vi "NI6071E_RT_Main.vi"(9 "Port":u16=6341) -> ()   [LabVIEW 2009]
uses:
  NI6071ECommand.ctl
  NI6071ECommandCluster.ctl
  NI6071EConfig.ctl
  NI6071EStart.ctl
  NI6071ERead.ctl
  <vilib>/Utility/error.llb/DialogType.ctl
  NI6071E.lvlib
panel:
  out "remote address":string
  in  "NI6071E DAQ Read":T1={"time limit in sec (-1:auto calculate)"=-1.0, "number of scans to read (-1:all)"=-1} {"time limit in sec (-1:auto calculate)" format="%0.2f"}
  in  "NI6071E DAQ Start":T2={"scan rate (40000 scans/sec)"=1000.0, "trigger type (analog)"=enum."no trigger", "edge or slope \n(rising)"=enum."no change", "number of buffers to acquire (1)"=1, "analog chan (PFI0) & level (2.00)"={"trigger channel (empty)"="", "level (0.0)"=0.0}, "[additional trig params]"={"hysteresis (0.0)"=-1.0, "coupling (no change:0)"=enum."no change", "delay (0 sec)"=0.0, "skip count (0)"=0, "time limit (0 sec)"=0.0}} {"[additional trig params]"."time limit (0 sec)" format="%0.2f"; "[additional trig params]"."delay (0 sec)" format="%0.2f"; "[additional trig params]"."hysteresis (0.0)" format="%0.2f"; "analog chan (PFI0) & level (2.00)"."level (0.0)" format="%0.2f"; "scan rate (40000 scans/sec)" format="%0.2f"}
  out "NI6071E DAQ Config":T3={"device (1)"=1, "channels (0)"=["0"], "buffer size (1000 scans)"=1000, "[number of buffers] (1)"=1, "measurement mode structure"={"measurement mode"=0, "reserved"=0}, "input limits (no change)"=[], "coupling & input config (no change:0)"=[]} {"measurement mode structure"."measurement mode" items=["no change", "Volts", "Volts RMS", "Ohms", "Diode", "4-wire ohms", "Current", "Current RMS"]; "coupling & input config (no change:0)"."input config (no change:0)" items=["no change", "differential", "ref. single-ended", "non-ref. single-ended", "4-wire"]; "input limits (no change)"."low limit (0.0)" format="%0.2f"; "input limits (no change)"."high limit (0.0)" format="%0.2f"}
  in  "NI6071E Config Default":T3={"device (1)"=1, "channels (0)"=["0"], "buffer size (1000 scans)"=1000, "[number of buffers] (1)"=1, "measurement mode structure"={"measurement mode"=0, "reserved"=0}, "input limits (no change)"=[], "coupling & input config (no change:0)"=[]} {"measurement mode structure"."measurement mode" items=["no change", "Volts", "Volts RMS", "Ohms", "Diode", "4-wire ohms", "Current", "Current RMS"]; "coupling & input config (no change:0)"."input config (no change:0)" items=["no change", "differential", "ref. single-ended", "non-ref. single-ended", "4-wire"]; "input limits (no change)"."low limit (0.0)" format="%0.2f"; "input limits (no change)"."high limit (0.0)" format="%0.2f"}
  in  "taskID in":u32 format="%x"
  out "Error string":string
  in  "NI6071E Command Cluster":T4
  out "Measurement":waveform(dbl)[](graph)
  out "NI6071E Command":T5=enum."ConfigureDAQ"
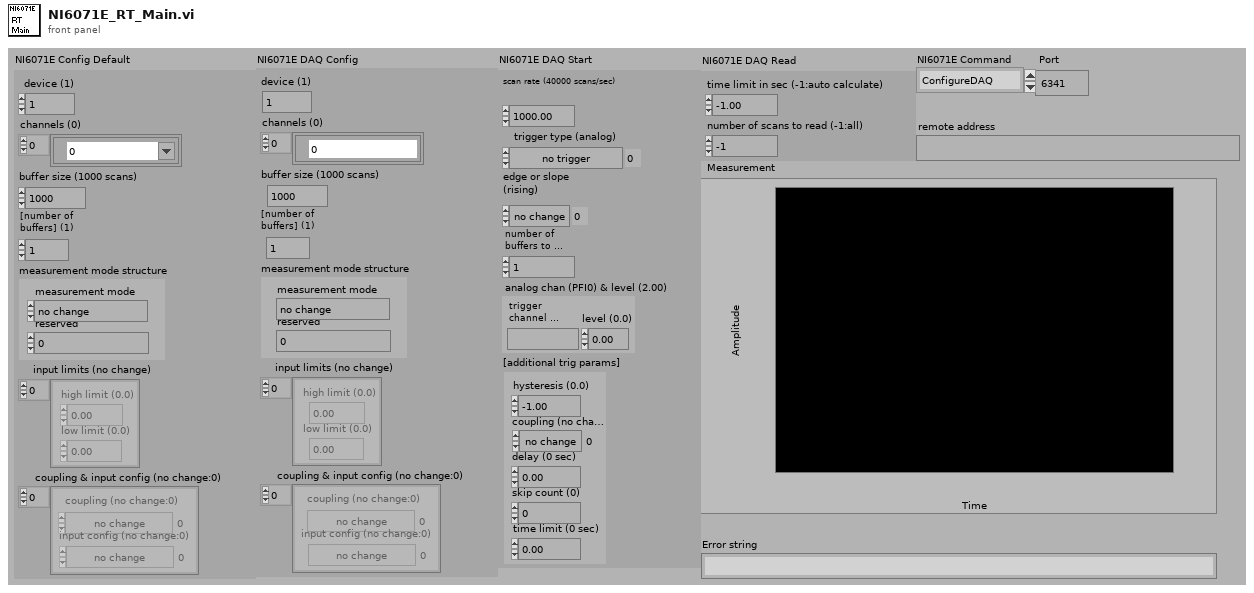
[diagram p1: front panel]
types:
  T1 = typedef "NI6071E.lvlib/NI6071ERead.ctl" = cluster{"time limit in sec (-1:auto calculate)":sgl, "number of scans to read (-1:all)":i32}
  T2 = typedef "NI6071E.lvlib/NI6071EStart.ctl" = cluster{"scan rate (40000 scans/sec)":sgl, "trigger type (analog)":enum16{"no trigger", "analog", "digital A", "digital A & B", "scan clock gate"}, "edge or slope \n(rising)":enum16{"no change", "rising", "falling"}, "number of buffers to acquire (1)":i32, "analog chan (PFI0) & level (2.00)":cluster{"trigger channel (empty)":string, "level (0.0)":sgl}, "[additional trig params]":cluster{"hysteresis (0.0)":sgl, "coupling (no change:0)":enum16{"no change", "DC", "AC"}, "delay (0 sec)":sgl, "skip count (0)":i32, "time limit (0 sec)":sgl}}
  T3 = typedef "NI6071E.lvlib/NI6071EConfig.ctl" = cluster{"device (1)":i16, "channels (0)":tag[], "buffer size (1000 scans)":i32, "[number of buffers] (1)":i32, "measurement mode structure":cluster{"measurement mode":u16, "reserved":u32}, "input limits (no change)":cluster{"high limit (0.0)":sgl, "low limit (0.0)":sgl}[], "coupling & input config (no change:0)":cluster{"coupling (no change:0)":enum16{"no change", "DC", "AC", "GND", "internal ref."}, "input config (no change:0)":u16}[]}
  T4 = typedef "NI6071E.lvlib/NI6071ECommandCluster.ctl" = cluster{"Command":string, "Data":string, "error out":errorcluster}
  T5 = typedef "NI6071E.lvlib/NI6071ECommand.ctl" = enum16{"Ping", "Reset", "ConfigureDAQ", "StartDAQ", "StopDAQ", "GetDAQStatus", "ReadData", "SaveData", "CloseConnection"}
  T6 = typedef "DialogType.ctl" = u16
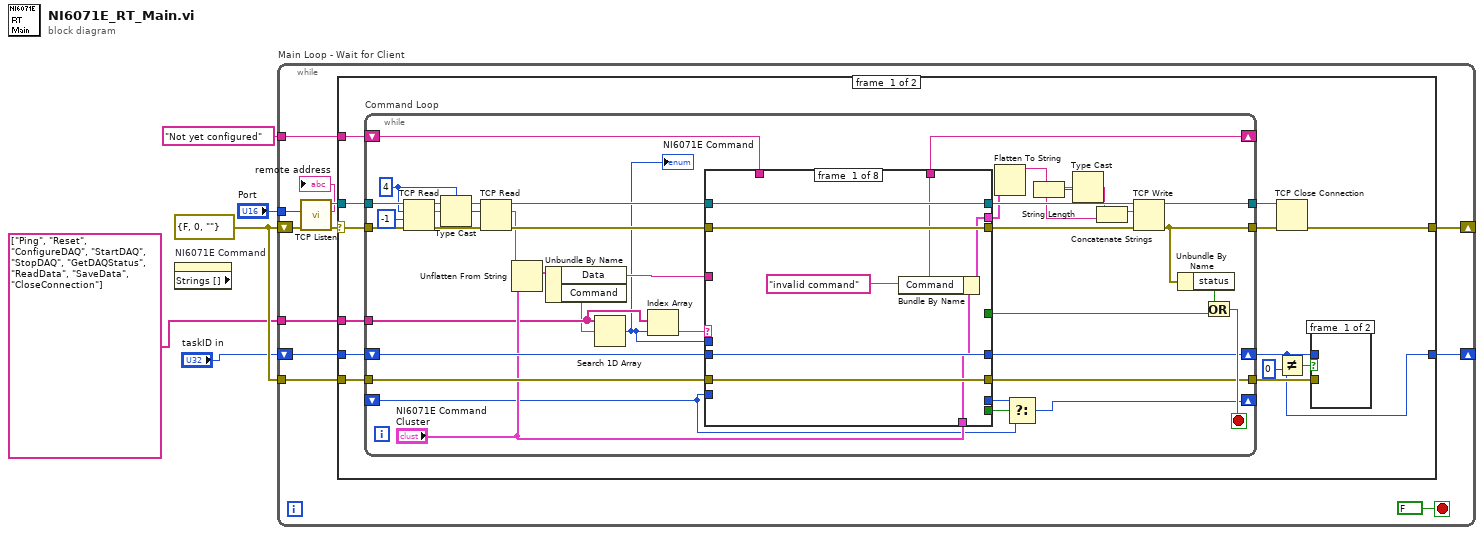
[diagram p0: block diagram]
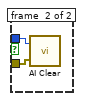
[diagram p2: hidden frame]
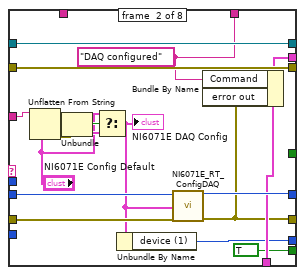
[diagram p3: hidden frame]
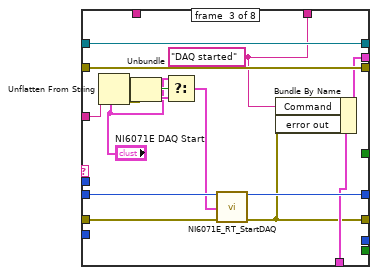
[diagram p4: hidden frame]
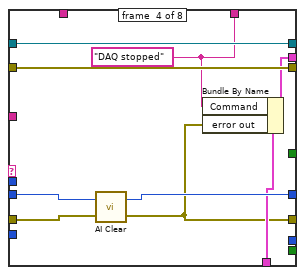
[diagram p5: hidden frame]
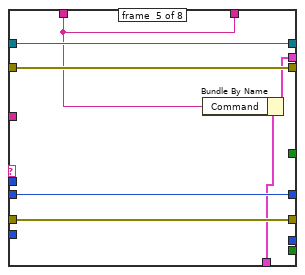
[diagram p6: hidden frame]
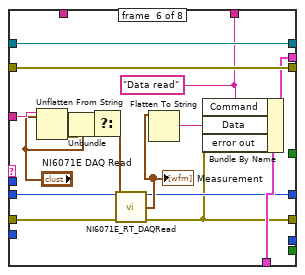
[diagram p7: hidden frame]
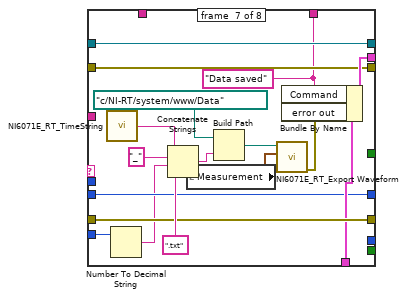
[diagram p8: hidden frame]
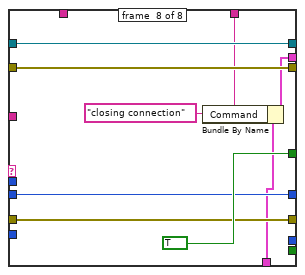
[diagram p9: hidden frame]
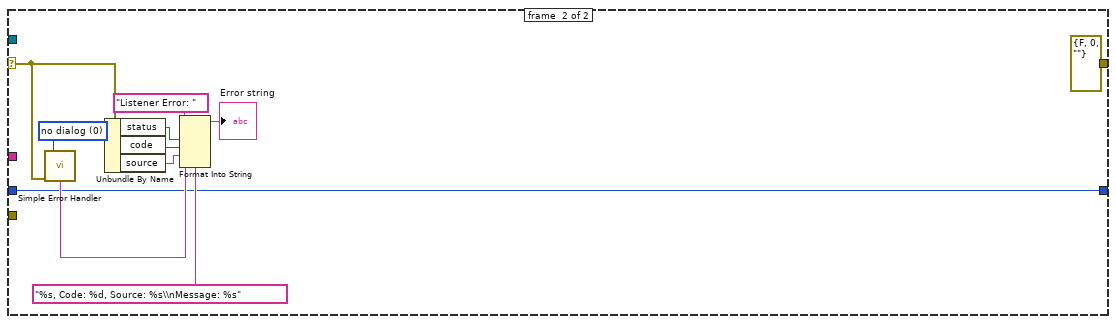
[diagram p10: hidden frame]
diagram:
  w5 = errorcluster {"status"=FALSE, "code"=0, "source"=""} ("error out")
  n1 = property on="NI6071E Command" class="Enum (strict)" props=["Strings []"]() -> ()  [unwired: 2 in, 3 out]
  n2 = while "Main Loop - Wait for Client" {
    tunnel: "Port" -> [w17]
    shift-right: [w12] -> _
    shift-left: w5 -> [w13]
    tunnel: string[] ["Ping", "Reset", "ConfigureDAQ", "StartDAQ", "StopDAQ", "GetDAQStatus", "ReadData", "SaveData", "CloseConnection"] ("Strings []") -> [w11]
    shift-right: [w9] -> _
    shift-left: "taskID in" -> [w10]
    tunnel: w5 -> [w8]
    tunnel: "Not yet configured" -> [w7]
    stop <- FALSE stop-if-true
    n3 = call <vilib>:"TCP Listen.vi"("error in (no error)"=w13, "port"=w17) -> ("error out"=w16:errorcluster, "remote address"=→"remote address":string, "connection ID"=w14:refnum<k5>)  [unwired: 6 in, 1 out]
    n4 = case shown="No Error" w16 {
      selector: w16 -> [w29 w173]
      tunnel: w14 -> [w30 _]
      tunnel: [w27 errorcluster {"status"=FALSE, "code"=0, "source"=""} ("error out")] -> w12
      tunnel: w11 -> [w25 _]
      tunnel: w10 -> [w24 w171]
      tunnel: [w19 w171] -> w9
      tunnel: w8 -> [w20 _]
      tunnel: w7 -> [w18 _]
      frame #0 {
        w19 = u32 0 ("taskID in")
        n5 = while "Command Loop" {
          tunnel: w30 -> [w72]
          tunnel: w29 -> [w71]
          tunnel: [w57] -> w28
          tunnel: [w58] -> w26
          tunnel: w25 -> [w36]
          tunnel: w20 -> [w46]
          tunnel: [w47] -> w21
          shift-right: [w51] -> w22
          shift-left: w24 -> [w52]
          shift-right: [w42] -> _
          shift-left: w18 -> [w41]
          shift-right: [w38] -> _
          shift-left: _ -> [w37]
          stop <- w61 stop-if-true
          w68 = 4 ("bytes to read")
          n6 = TCP Read(connection ID=w72, bytes to read=w68, error in (no error)=w71, 9:-1 ("timeout ms (25000)")) -> (connection ID out=w67:refnum<k5>, data out=w69:string, error out=w66:errorcluster)  [unwired: 1 in]
          n7 = Type Cast(type=w68, x=w69) -> (*(type *) &x=w53:i32)
          n8 = TCP Read(connection ID=w67, bytes to read=w53, error in (no error)=w66) -> (connection ID out=w64:refnum<k5>, data out=w49:string, error out=w65:errorcluster)  [unwired: 2 in]
          n9 = Unflatten From String(type="NI6071E Command Cluster", binary string=w49) -> (value=w50:T4)  [unwired: 3 in, 2 out]
          n10 = Unbundle By Name(w50) -> ("Data"=w48:string, "Command"=w34:string)
          n11 = Search 1D Array(1D array=w36, element=w34) -> (index of element=w35:i32)  [unwired: 1 in]
          "NI6071E Command" <- w35
          n12 = Index Array(array=w36, index=w35) -> (element=w33:string)
          n13 = case shown="\"ConfigureDAQ\"" w33 {
            tunnel: [_ _ _ _ _ _ _ TRUE] -> w62
            tunnel: w65 -> [w78 w92 w107 w117 w126 w143 w150 w167]
            tunnel: w64 -> [w79 w96 w111 w120 w127 w144 w161 w168]
            tunnel: [w79 w96 w111 w120 w127 w144 w161 w168] -> w59
            tunnel: [w78 w92 w107 w117 w126 w143 w150 w167] -> w60
            tunnel: [w74 w86 w105 w114 w122 w138 w152 w163] -> w44
            tunnel: w52 -> [w77 w91 w110 w119 w125 w129 w147 w166]
            tunnel: [w77 w90 w109 w118 w125 w134 w147 w166] -> w51
            tunnel: w48 -> [_ w95 w100 _ _ w140 _ _]
            tunnel: [w76 w85 w104 w113 w124 w133 w154 w165] -> w47
            tunnel: w46 -> [w76 w89 w108 w116 w124 w132 w154 w165]
            tunnel: "NI6071E Command Cluster" -> [w75 w87 w106 w115 w123 w137 w153 w164]
            tunnel: [w73 w84 w98 w112 w121 w136 w149 w162] -> w42
            tunnel: w41 -> [_ _ _ _ w121 _ _ _]
            tunnel: [_ w82 _ _ _ _ _ _] -> w40
            tunnel: [_ TRUE _ _ _ _ _ _] -> w39
            tunnel: w37 -> [_ _ _ _ _ _ w146 _]
            tunnel: w35 -> [_ _ _ _ _ _ _ _]
            frame #0 {
              w73 = "invalid command"
              n14 = Bundle By Name(cluster=w75, "Command"=w73) -> (w74:T4)
            }
            frame #1 {
              w84 = "DAQ configured"
              n15 = Unflatten From String(type="NI6071E Config Default", binary string=w95) -> (value=w93:T3, error out=w80:errorcluster)  [unwired: 3 in, 1 out]
              n16 = Unbundle(w80) -> ("status"=w94:bool)  [unwired: 2 out]
              n17 = Select(t="NI6071E Config Default", s=w94, f=w93) -> (s? t:f=w83:T3)
              "NI6071E DAQ Config" <- w83
              n18 = Unbundle By Name(w83) -> ("device (1)"=w82:i16)
              n19 = call "NI6071E_RT_ConfigDAQ.vi"("taskID in"=w91, "NI6071E DAQ Config"=w83, "error in (no error)"=w89) -> ("taskID out"=w90:u32, "error out"=w85:errorcluster)  [unwired: 10 in, 1 out]
              n20 = Bundle By Name(cluster=w87, "Command"=w84, "error out"=w85) -> (w86:T4)
            }
            frame #2 {
              w98 = "DAQ started"
              n21 = Unflatten From String(type="NI6071E DAQ Start", binary string=w100) -> (value=w102:T2, error out=w97:errorcluster)  [unwired: 3 in, 1 out]
              n22 = Unbundle(w97) -> ("status"=w103:bool)  [unwired: 2 out]
              n23 = Select(t="NI6071E DAQ Start", s=w103, f=w102) -> (s? t:f=w99:T2)
              n24 = call "NI6071E_RT_StartDAQ.vi"("taskID in"=w110, "NI6071E DAQ Start"=w99, "error in"=w108) -> ("taskID out"=w109:u32, "error out"=w104:errorcluster)  [unwired: 11 in]
              n25 = Bundle By Name(cluster=w106, "Command"=w98, "error out"=w104) -> (w105:T4)
            }
            frame #3 {
              w112 = "DAQ stopped"
              n26 = call <vilib>:"AI Clear.vi"("error in (no error)"=w116, "taskID in"=w119) -> ("error out"=w113:errorcluster, "taskID out"=w118:u32)  [unwired: 4 in]
              n27 = Bundle By Name(cluster=w115, "Command"=w112, "error out"=w113) -> (w114:T4)
            }
            frame #4 {
              n28 = Bundle By Name(cluster=w123, "Command"=w121) -> (w122:T4)
            }
            frame #5 {
              w136 = "Data read"
              n29 = Unflatten From String(type="NI6071E DAQ Read", binary string=w140) -> (value=w141:T1, error out=w128:errorcluster)  [unwired: 3 in, 1 out]
              n30 = Unbundle(w128) -> ("status"=w142:bool)  [unwired: 2 out]
              n31 = Select(t="NI6071E DAQ Read", s=w142, f=w141) -> (s? t:f=w130:T1)
              n32 = call "NI6071E_RT_DAQRead.vi"("taskID in"=w129, "NI6071E Read"=w130, "error in"=w132) -> ("taskID out"=w134:u32, "Measurement"=w135:waveform(dbl)[], "error out"=w133:errorcluster)  [unwired: 10 in]
              "Measurement" <- w135
              n33 = Flatten To String(anything=w135) -> (data string=w139:string)  [unwired: 3 in, 2 out]
              n34 = Bundle By Name(cluster=w137, "Command"=w136, "Data"=w139, "error out"=w133) -> (w138:T4)
            }
            frame #6 {
              w149 = "Data saved"
              n35 = call "NI6071E_RT_TimeString.vi"() -> ("date/time string"=w157:string)
              n36 = Number To Decimal String(number=w146) -> (decimal integer string=w145:string)  [unwired: 1 in]
              n37 = Concatenate Strings(w157, "_" ("string"), w145, ".txt" ("string")) -> (w155:string)
              n38 = local read "Measurement"() -> (w160:waveform(dbl)[])
              n39 = Build Path(base path=path "c:/NI-RT/system/www/Data" ("file path (dialog if empty)"), name or relative path=w155) -> (appended path=w158:path)
              n40 = call "NI6071E_RT_Export Waveform.vi"("Waveforms"=w160, "file path (dialog if empty)"=w158) -> ("error out"=w151:errorcluster)  [unwired: 8 in, 1 out]
              n41 = Bundle By Name(cluster=w153, "Command"=w149, "error out"=w151) -> (w152:T4)
            }
            frame #7 {
              w162 = "closing connection"
              n42 = Bundle By Name(cluster=w164, "Command"=w162) -> (w163:T4)
            }
          }
          n43 = Flatten To String(anything=w44) -> (data string=w45:string)  [unwired: 3 in, 2 out]
          n44 = Select(t=w40, s=w39, f=w37) -> (s? t:f=w38:i16)
          n45 = String Length(string=w45) -> (length=w54:i32)
          n46 = Type Cast(type=w45, x=w54) -> (*(type *) &x=w55:string)
          n47 = Concatenate Strings(w55, w45) -> (w56:string)
          n48 = TCP Write(connection ID=w59, data in=w56, error in (no error)=w60) -> (connection ID out=w57:refnum<k5>, error out=w58:errorcluster)  [unwired: 1 in, 1 out]
          n49 = Unbundle By Name(w58) -> ("status"=w63:bool)
          n50 = Or(x=w63, y=w62) -> (x .or. y?=w61:bool)
        }
        n51 = TCP Close Connection(connection ID=w28, error in (no error)=w26) -> (error out=w27:errorcluster)  [unwired: 1 in, 1 out]
        n52 = Not Equal?(x=w22, y=w19) -> (x != y?=w23:bool)
        n53 = case shown="True" w23 {
          tunnel: w22 -> [_ w31]
          tunnel: w21 -> [_ w32]
          frame #0 {
          }
          frame #1 {
            n54 = call <vilib>:"AI Clear.vi"("error in (no error)"=w32, "taskID in"=w31) -> ()  [unwired: 4 in, 2 out]
          }
        }
      }
      frame #1 {
        w175 = T6 0 items=["no dialog", "OK message", "continue or stop message", "OK message + warnings", "continue/stop + warnings"] ("type of dialog (OK msg:1)")
        n55 = call <vilib>:"Simple Error Handler.vi"("type of dialog (OK msg:1)"=w175, "error in (no error)"=w173) -> ("message"=w174:string)  [unwired: 3 in, 4 out]
        n56 = Unbundle By Name(w173) -> ("status"=w180:bool, "code"=w179:i32, "source"=w178:string)
        n57 = Format Into String(format string="%s, Code: %d, Source: %s\\nMessage: %s", initial string="Listener Error: ", w180, w179, w178, w174) -> (resulting string=→"Error string":string)  [unwired: 1 in, 1 out]
      }
    }
  }
